vi "StraightDrive.vi"(9 "RightDrive in":dbl, 10 "LeftDrive in":dbl, 11 "StraightDrive":bool) -> (1 "RightDrive out":dbl, 2 "LeftDrive out":dbl)   [LabVIEW 2013]
doc: "When StraightDrive is true, takes the left joystick value and makes that both the left and right joystick values. Otherwise, no action is taken."
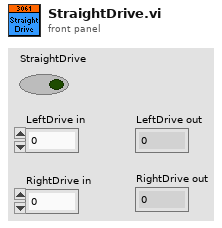
[diagram p1: front panel]
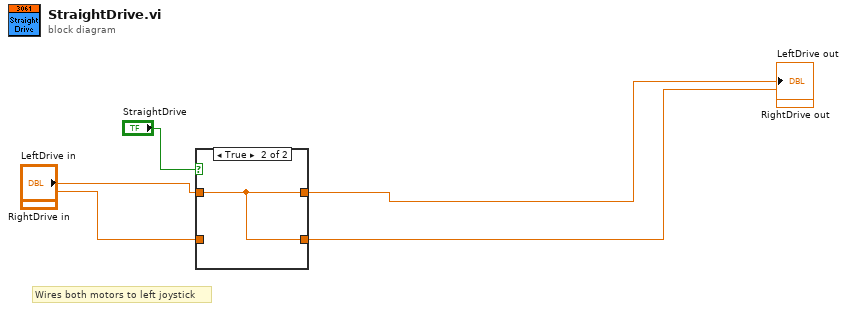
[diagram p0: block diagram]
diagram:
  # "Wires both motors to left joystick"
  n1 = case shown="True" "StraightDrive" {
    tunnel: [w7 w8] -> w4
    tunnel: "RightDrive in" -> [w7 _]
    tunnel: [w6 w8] -> w5
    tunnel: "LeftDrive in" -> [w6 w8]
    frame False {
    }
    frame True {
    }
  }
  "LeftDrive out" <- w5
  "RightDrive out" <- w4
